vi "Initalise_Bike_Parameter.vi"(8 "Ts":dbl=8.0 format="%#_13g", 9 "Velocity":dbl=8.0 format="%#_13g") -> (0 "Other variables":T1, 1 "systems":T6 {"SysD"."Transport Delay" format="%.2f"; "SysD"."D" format="%#.2g"; "SysD"."C" format="%#.2g"; "SysD"."B" format="%#.2g"; "SysD"."A" format="%#.2g"; "SysD"."properties"."Sampling Time" format="%#.6p"; "SysD"."properties"."Output Delays" format="%.4f"; "SysD"."properties"."Input Delays" format="%.4f"; "sysDo"."Transport Delay" format="%.2f"; "sysDo"."D" format="%#.2g"; "sysDo"."C" format="%#.2g"; "sysDo"."B" format="%#.2g"; "sysDo"."A" format="%#.2g"; "sysDo"."properties"."Sampling Time" format="%#.6p"; "sysDo"."properties"."Output Delays" format="%.4f"; "sysDo"."properties"."Input Delays" format="%.4f"; "sysDi"."Transport Delay" format="%.2f"; "sysDi"."D" format="%#.2g"; "sysDi"."C" format="%#.2g"; "sysDi"."B" format="%#.2g"; "sysDi"."A" format="%#.2g"; "sysDi"."properties"."Sampling Time" format="%#.6p"; "sysDi"."properties"."Output Delays" format="%.4f"; "sysDi"."properties"."Input Delays" format="%.4f"; "sysDC"."transfer function(s)"."delay" format="%.4f"; "sysDC"."transfer function(s)"."Denominator" format="%#_3g"; "sysDC"."transfer function(s)"."Numerator" format="%#_3g"; "sysDC"."properties"."Sampling Time" format="%#.6p"; "sysDC"."properties"."Output Delays" format="%.4f"; "sysDC"."properties"."Input Delays" format="%.4f"})   [LabVIEW 2016]
uses:
  <vilib>/addons/Control Design/_Model Construction/Model Typedefs.llb/CD State Space Model (MIMO).ctl
  <vilib>/addons/Control Design/_Model Construction/Model Typedefs.llb/CD General Elements.ctl
  <vilib>/addons/Control Design/_Model Construction/Model Typedefs.llb/CD Transfer Function Model (MIMO).ctl
  <vilib>/addons/Control Design/_Model Construction/Model Typedefs.llb/CD Transfer Function Model (SISO).ctl
  <vilib>/imath/engines/lvmath2/RunTimeEngine/Managers/WorkSpace/UID Generator.vi
  <vilib>/imath/engines/lvmath2/RunTimeEngine/BuiltInFunctions/deg_to_rad/NIMS_deg_to_rad.vi
  <instcachedir>/0/NIMS_deg_to_rad_4A81D684CE8D4DD79924F5AB74D756E1.lvgen/NIMS_deg_to_rad_4A81D684CE8D4DD79924F5AB74D756E1_001.vi
  <vilib>/imath/engines/lvmath2/RunTimeEngine/BuiltInFunctions/inv/NIMS_inv(GM).vi
  <instcachedir>/0/NIMS_inv(GM)_A6DF8FE880224208AACFE4CF9F659502.lvgen/NIMS_inv(GM)_A6DF8FE880224208AACFE4CF9F659502_000.vi
  <vilib>/imath/engines/lvmath2/RunTimeEngine/ArithmeticOperatorToken/NIMS_ArithmeticOperator_multmx.vi
  <instcachedir>/0/NIMS_ArithmeticOperator_multmx_4A56FE5C615140CE835D4DB5891BF065.lvgen/NIMS_ArithmeticOperator_multmx_4A56FE5C615140CE835D4DB5891BF065_004.vi
  <vilib>/imath/engines/lvmath2/RunTimeEngine/ErrorHandling/NIMS_Create Error From Enums.vi
  <vilib>/imath/engines/lvmath2/RunTimeEngine/RowToken/NIMS_RowToken_M_M.vi
  <instcachedir>/0/NIMS_RowToken_M_M_968CDE3545E74ACDAEA4B48DE01EEECA.lvgen/NIMS_RowToken_M_M_968CDE3545E74ACDAEA4B48DE01EEECA_005.vi
  <instcachedir>/0/NIMS_RowToken_M_M_968CDE3545E74ACDAEA4B48DE01EEECA.lvgen/NIMS_RowToken_M_M_968CDE3545E74ACDAEA4B48DE01EEECA_004.vi
  <vilib>/imath/engines/lvmath2/RunTimeEngine/MatrixToken/NIMS_MatrixToken_M_M.vi
  <instcachedir>/0/NIMS_MatrixToken_M_M_DF273B0CC20F424BBF1EDA9F4E71C841.lvgen/NIMS_MatrixToken_M_M_DF273B0CC20F424BBF1EDA9F4E71C841_004.vi
  <vilib>/imath/engines/lvmath2/RunTimeEngine/ArithmeticOperatorToken/NIMS_ArithmeticOperator_multmx(M,CV).vi
  <instcachedir>/0/NIMS_ArithmeticOperator_multmx(M,CV)_EE734FC8520844C9A7CC1A67008668A3.lvgen/NIMS_ArithmeticOperator_multmx(M,CV)_EE734FC8520844C9A7CC1A67008668A3_002.vi
  <vilib>/imath/engines/lvmath2/RunTimeEngine/MatrixToken/NIMS_MatrixToken_SorCV_M.vi
  <instcachedir>/0/NIMS_MatrixToken_SorCV_M_667D6DA9EAAA4E73AD685CBB2779BCDB.lvgen/NIMS_MatrixToken_SorCV_M_667D6DA9EAAA4E73AD685CBB2779BCDB_000.vi
  <vilib>/imath/engines/lvmath2/RunTimeEngine/RowToken/NIMS_RowToken_CV_CV.vi
  <instcachedir>/0/NIMS_RowToken_CV_CV_5546A0B1CA2C4E49826F811B9C073FB0.lvgen/NIMS_RowToken_CV_CV_5546A0B1CA2C4E49826F811B9C073FB0_000.vi
  <vilib>/imathl/engines/lvmath/Functions/Error Handling/Create Error.vi
  <vilib>/imath/engines/lvmath/Plug In/Control Design/BuiltInFunctions/ss/NIMS_CD_ss(A,B,C,D).vi
  <vilib>/imath/engines/lvmath/Plug In/Control Design/BuiltInFunctions/c_to_d/NIMS_CD_c_to_d(SS,TS,STR,DBL).vi
  <vilib>/imath/engines/lvmath2/RunTimeEngine/RunTimeType/NIMS_RunTimeType_From StrictType (excl LVString).vi
  <instcachedir>/0/NIMS_RunTimeType_From StrictType (excl LVString)_BBF44FB49F834B71AF7A14CCEDF8BECD.lvgen/NIMS_RunTimeType_From StrictType (excl LVString)_BBF44FB49F834B71AF7A14CCEDF8BECD_031.vi
  <vilib>/imath/engines/lvmath2/RunTimeEngine/LocalVariableDefStatement/MC_LocalVariableDefStatement_Display.vi
  <vilib>/imath/engines/lvmath2/RunTimeEngine/ErrorHandling/NIMS_Error From Error Code.vi
  <vilib>/imath/engines/lvmath2/RunTimeEngine/IndexRead/NIMS M(S,S).vi
  <instcachedir>/0/NIMS M(S,S)_AC51E74150A542F7991B9634C66F3096.lvgen/NIMS M(S,S)_AC51E74150A542F7991B9634C66F3096_000.vi
  <instcachedir>/0/NIMS_RunTimeType_From StrictType (excl LVString)_BBF44FB49F834B71AF7A14CCEDF8BECD.lvgen/NIMS_RunTimeType_From StrictType (excl LVString)_BBF44FB49F834B71AF7A14CCEDF8BECD_000.vi
  <vilib>/imath/engines/lvmath/Plug In/Control Design/BuiltInFunctions/tf/NIMS_CD_tf(num,den,Ts).vi
  <vilib>/imath/engines/lvmath/Plug In/Control Design/BuiltInFunctions/c_to_d/NIMS_CD_c_to_d(TF,TS,STR,DBL).vi
  <vilib>/imath/engines/lvmath2/RunTimeEngine/Managers/SymbolTable/Clear UID.vi
  <vilib>/imath/engines/lvmath2/RunTimeEngine/NodeEndStatement/NIMS_NodeEndStatement_Output.vi
  <instcachedir>/0/NIMS_NodeEndStatement_Output_53EC0D466D134D7ABD903AC30B43404B.lvgen/NIMS_NodeEndStatement_Output_53EC0D466D134D7ABD903AC30B43404B_005.vi
  <instcachedir>/0/NIMS_NodeEndStatement_Output_53EC0D466D134D7ABD903AC30B43404B.lvgen/NIMS_NodeEndStatement_Output_53EC0D466D134D7ABD903AC30B43404B_011.vi
  <instcachedir>/0/NIMS_NodeEndStatement_Output_53EC0D466D134D7ABD903AC30B43404B.lvgen/NIMS_NodeEndStatement_Output_53EC0D466D134D7ABD903AC30B43404B_010.vi
  <instcachedir>/0/NIMS_NodeEndStatement_Output_53EC0D466D134D7ABD903AC30B43404B.lvgen/NIMS_NodeEndStatement_Output_53EC0D466D134D7ABD903AC30B43404B_001.vi
  <instcachedir>/0/NIMS_NodeEndStatement_Output_53EC0D466D134D7ABD903AC30B43404B.lvgen/NIMS_NodeEndStatement_Output_53EC0D466D134D7ABD903AC30B43404B_002.vi
  <vilib>/imath/engines/lvmath2/RunTimeEngine/ErrorHandling/NIMS_Finalize Error.vi
  <vilib>/imath/engines/lvmath2/RunTimeEngine/Managers/SymbolTable/NIMS_WorkSpace.lvlib
  <vilib>/addons/Control Design/_Model Construction/NI_LinSys_Model Typedefs.lvlib
panel:
  out "Lo":dbl[][](array[numeric])
  # "Inputs"
  # "Outputs"
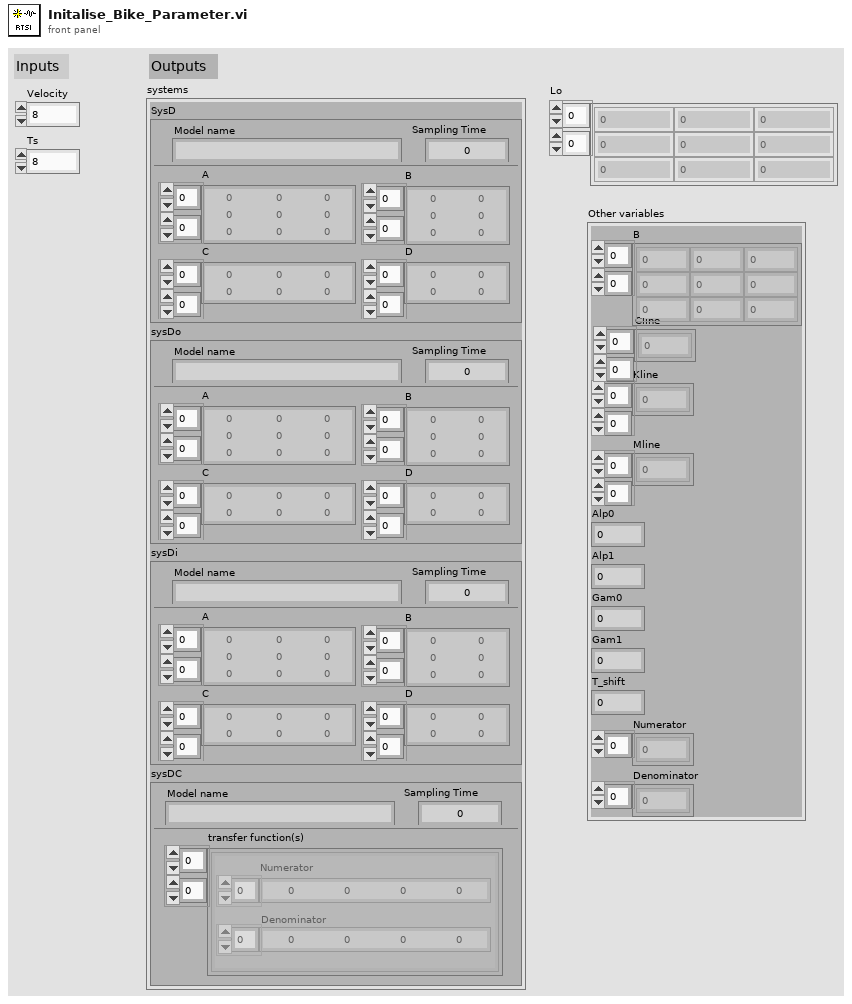
[diagram p1: front panel]
types:
  T1 = cluster{"B":dbl[][], "Cline":dbl[][], "Kline":dbl[][], "Mline":dbl[][], "Alp0":dbl, "Alp1":dbl, "Gam0":dbl, "Gam1":dbl, "T_shift":dbl, "Numerator":dbl[], "Denominator":dbl[]}
  T2 = typedef "NI_LinSys_Model Typedefs.lvlib/CD State Space Model (MIMO).ctl" = cluster{"properties":T3, "A":dbl[][], "B":dbl[][], "C":dbl[][], "D":dbl[][], "StateNames":string[], "Transport Delay":dbl[][]}
  T3 = typedef "NI_LinSys_Model Typedefs.lvlib/CD General Elements.ctl" = cluster{"Model name":string, "Input names":string[], "Output names":string[], "Input Delays":dbl[], "Output Delays":dbl[], "Sampling Time":dbl, "Notes":string}
  T4 = typedef "NI_LinSys_Model Typedefs.lvlib/CD Transfer Function Model (MIMO).ctl" = cluster{"properties":T3, "transfer function(s)":T5[][]}
  T5 = typedef "NI_LinSys_Model Typedefs.lvlib/CD Transfer Function Model (SISO).ctl" = cluster{"Numerator":dbl[], "Denominator":dbl[], "delay":dbl}
  T6 = cluster{"SysD":T2, "sysDo":T2, "sysDi":T2, "sysDC":T4}
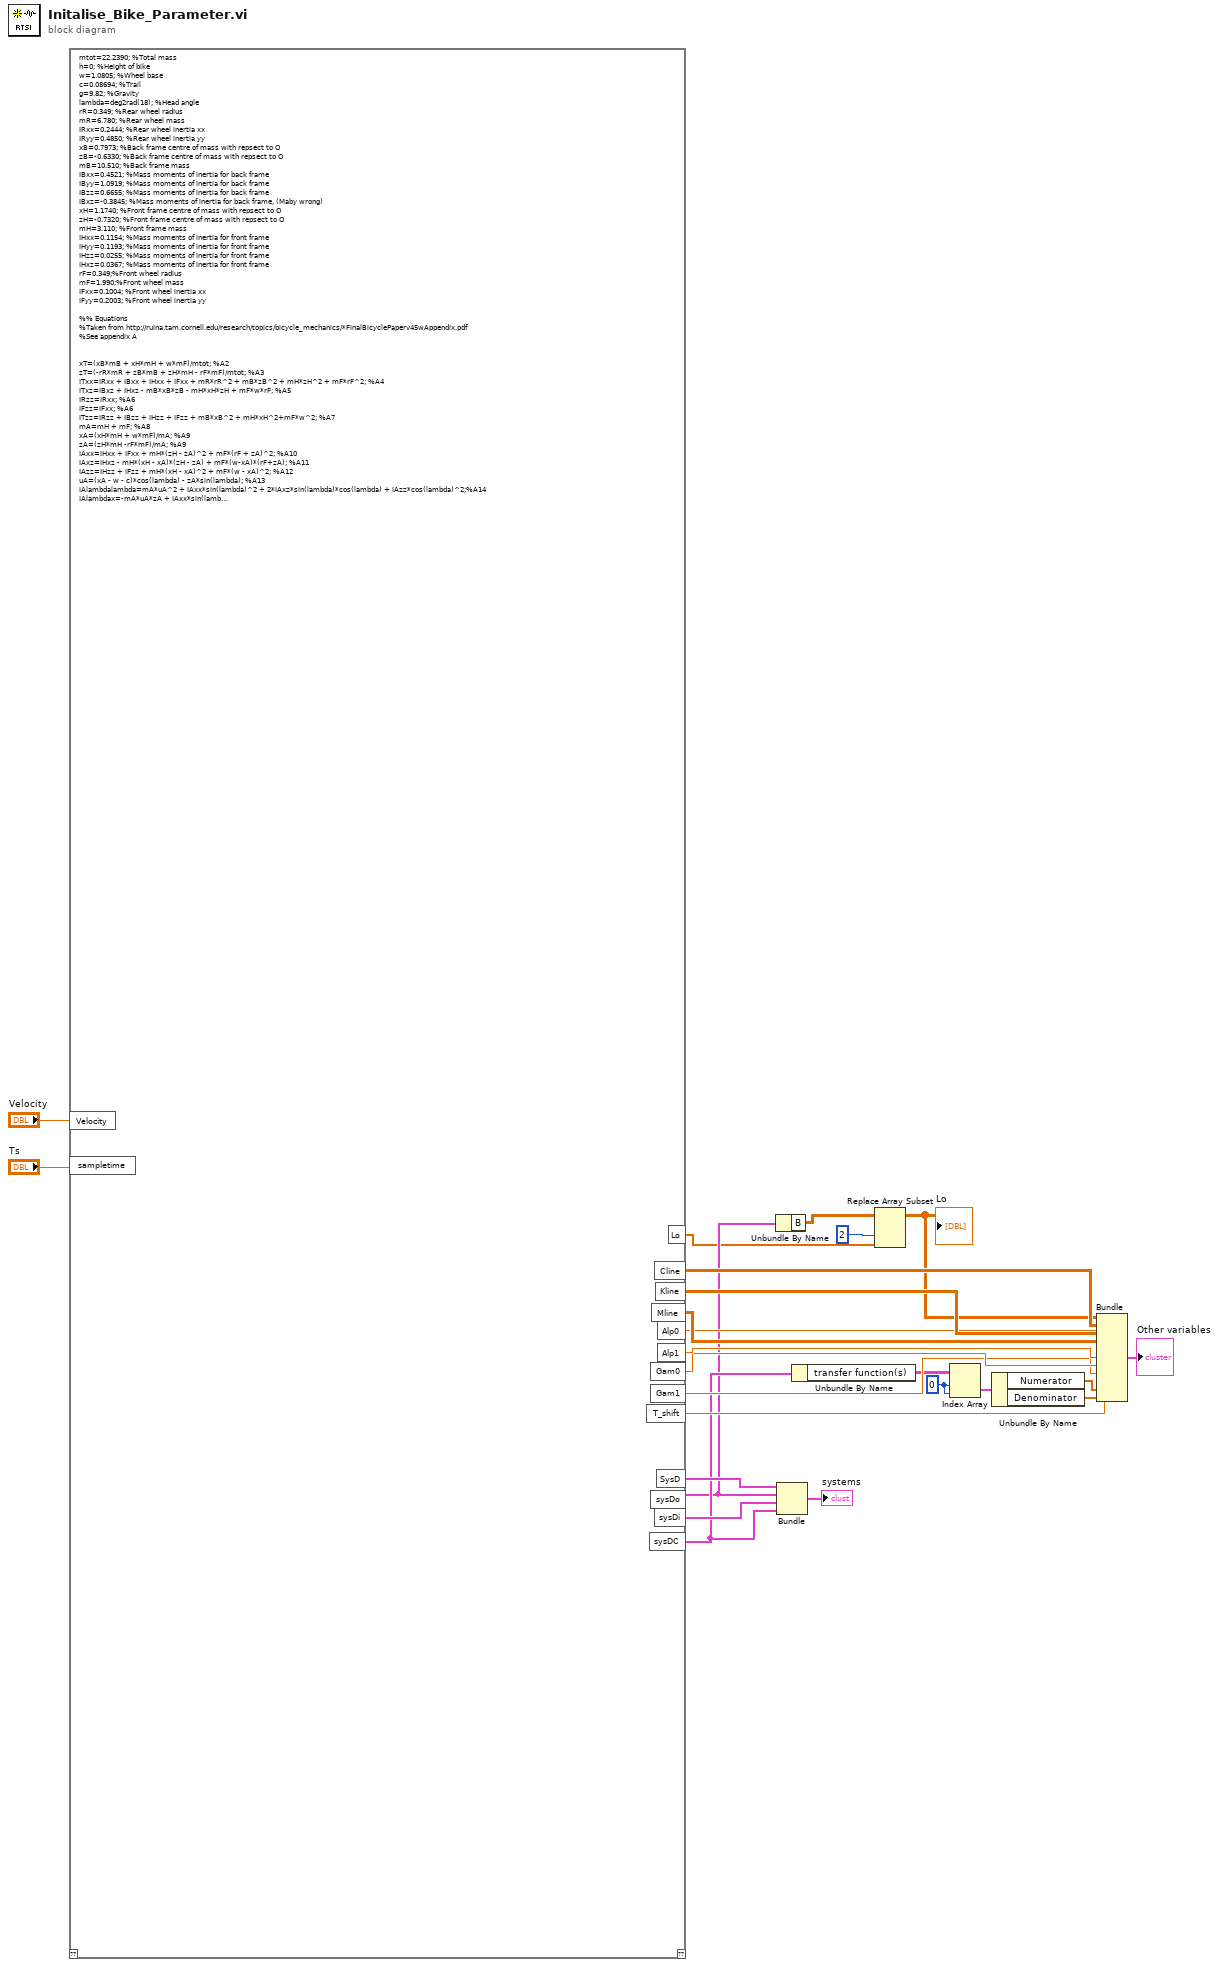
[diagram p0: block diagram]
diagram:
  w12 = 0 ("index (row)")
  n1 = mathscript code="mtot=22.2390; %Total mass\nh=0; %Height of bike\nw=1.0805; %Wheel base\nc=0.08694; %Trail\ng=9.82; %Gravity\nlambda=deg2rad(18); %Head angle\nrR=0.349; %Rear wheel radius\nmR=6.780; %Rear wheel mass\nIRxx=0.2444; %Rear wheel inertia xx\nIRyy=0.4850; %Rear wheel inertia yy\nxB=0.7973; %Back frame centre of mass with repsect to O\nzB=-0.6330; %Back frame centre of mass with repsect to O\nmB=10.510; %Back frame mass\nIBxx=0.4521; %Mass moments of inertia for back frame\nIByy=1.0919; %Mass moments of inertia for back frame\nIBzz=0.6655; %Mass moments of inertia for back frame\nIBxz=-0.3845; %Mass moments of inertia for back frame, (Maby wrong)\nxH=1.1740; %Front frame centre of mass with repsect to O\nzH=-0.7320; %Front frame centre of mass with repsect to O\nmH=3.110; %Front frame mass\nIHxx=0.1154; %Mass moments of inertia for front frame\nIHyy=0.1193; %Mass moments of inertia for front frame\nIHzz=0.0255; %Mass moments of inertia for front frame\nIHxz=0.0367; %Mass moments of inertia for front frame\nrF=0.349;%Front wheel radius\nmF=1.990;%Front wheel mass\nIFxx=0.1004; %Front wheel inertia xx\nIFyy=0.2003; %Front wheel inertia yy \n\n%% Equations\n%Taken from http://ruina.tam.cornell.edu/research/topics/bicycle_mechanics/*FinalBicyclePaperv45wAppendix.pdf\n%See appendix A\n\n\nxT=(xB*mB + xH*mH + w*mF)/mtot; %A2\nzT=(-rR*mR + zB*mB + zH*mH - rF*mF)/mtot; %A3\nITxx=IRxx + IBxx + IHxx + IFxx + mR*rR^2 + mB*zB^2 + mH*zH^2 + mF*rF^2; %A4\nITxz=IBxz + IHxz - mB*xB*zB - mH*xH*zH + mF*w*rF; %A5\nIRzz=IRxx; %A6\nIFzz=IFxx; %A6\nITzz=IRzz + IBzz + IHzz + IFzz + mB*xB^2 + mH*xH^2+mF*w^2; %A7\nmA=mH + mF; %A8\nxA=(xH*mH + w*mF)/mA; %A9\nzA=(zH*mH -rF*mF)/mA; %A9\nIAxx=IHxx + IFxx + mH*(zH - zA)^2 + mF*(rF + zA)^2; %A10\nIAxz=IHxz - mH*(xH - xA)*(zH - zA) + mF*(w-xA)*(rF+zA); %A11\nIAzz=IHzz + IFzz + mH*(xH - xA)^2 + mF*(w - xA)^2; %A12\nuA=(xA - w - c)*cos(lambda) - zA*sin(lambda); %A13\nIAlambdalambda=mA*uA^2 + IAxx*sin(lambda)^2 + 2*IAxz*sin(lambda)*cos(lambda) + IAzz*cos(lambda)^2;%A14\nIAlambdax=-mA*uA*zA + IAxx*sin(lambda) + IAxz*cos(lambda); %A15\nIAlambdaz=mA*uA*xA + IAxz*sin(lambda) + IAzz*cos(lambda); %A16\nmy=(c/w)*cos(lambda); %A17\nSR=IRyy/rR; %A18\nSF=IFyy/rF; %A18\nST=SR + SF; %A18\nSA=mA*uA + my*mtot*xT; %A19\nMfifi=ITxx; %A20\nMfidelta=IAlambdax + my*ITxz; %A20\nMdeltadelta=IAlambdalambda + 2*my*IAlambdaz + my^2*ITzz; %A20\nM=[Mfifi Mfidelta; Mfidelta Mdeltadelta]; %A21r\nK0fifi=mtot*zT; %A22\nK0fidelta=-SA; %A22\nK0deltadelta=-SA*sin(lambda); %A22\nK0=[K0fifi K0fidelta; K0fidelta K0deltadelta]; %A23\nK2fifi=0; %A24\nK2fidelta=((ST - mtot*zT)/w)*cos(lambda); %A24\nK2deltafi=0; %A24\nK2deltadelta=((SA + SF*sin(lambda))/w)*cos(lambda); %A24\nK2=[K2fifi K2fidelta; K2deltafi K2deltadelta]; %A25\nC1fifi=0; %A26\nC1fidelta=my*ST + SF*cos(lambda) + (ITxz/w)*cos(lambda) - my*mtot*zT; %A26\nC1deltafi=-(my*ST + SF*cos(lambda)); %A26\nC1deltadelta=(IAlambdaz/w)*cos(lambda) + my*(SA + (ITzz/w)*cos(lambda)); %A26\nC1=[C1fifi C1fidelta; C1deltafi C1deltadelta]; %A27\n %C=v*C1;\n Ts=sampletime;\n\n \n %%  Wipple model \n %A matrix\n v=Velocity/3.6;\n A1=[0 0; 0 0];\n A2=[1 0; 0 1];\n A3=-inv(M)*(g*K0+v^2*K2);\n A4=-inv(M)*v*C1;\n A=[A1, A2; A3, A4];\n \n %B matrix\n B=[[0; 0]; inv(M)*[0;1]]; \n %B1 matrix\n B1=[[0; 0]; inv(M)*[1;0]]; \n %C matrix\n C=[1 0 0 0; 0 1 0 0];\n %D matrix\n D=[0 0; 0 0];\n\nsys = ss(A, [B B1],C, D); \nSysD= c2d(sys,Ts)\n %% Lean angle control loop\n Cline=v*inv(M)*C1;\n Kline=inv(M)*(g*K0+v^2*K2);\n Mline=inv(M);\n\n%duty cycle constant\nKt=0.0273;\nKe=24/100;\nRm=0.33;\n\nDutyCycleTransform=0.009/((Mline(2,2)*Kt*Ke)/Rm); %duty cycle conversion \nT_shift=DutyCycleTransform; %torque conversion \n\n% Alpha and Gamma\nAlp1=4.367;\nAlp0=22.812\n\nGam1=38.538;\nGam0=448.438;\n\n \n%Outer control loop - stabilizing controller\n \nAo=[0 1 0; -Kline(1,1) -Cline(1,1) 1; 0 0 0]; %d \nBo=[0 0 1.557*10^3 ; 1 Mline(1,2) 5.386*10^5; 0 0 4.148*10^7]; \nCo=[1 0 0]; %f\nDo=[0 0 0]; %f\nLo=[2.097 257.5 1.346e+04]'\n \nsyso=ss(Ao,Bo,Co,Do);\nsysDo=c2d(syso, Ts);\n\n% modfi L gains \n%Lo=[2.097; 257.5 ;1.346e+04];\n%sysDo.B(:,3)=Lo;\n%Inner control loop - stabilizing controller\n \nAi=[0 1 0 0 0 0; -Kline(2,2) -Cline(2,2) 1 0 0 0; 0 0 0 1 0 0; 0 0 0 0 1 0; 0 0 0 0 0 1; 0 0 0 0 0 0];\nBi=[ 0 0 0 1.099*10^2; Mline(2,2) -Cline(2,1) -Kline(2,1) 4.693*10^3; 0  0  0 1.094*10^5;  0 0 0 0.22*10^5; 0 0 0 0.22*10^4; 0 0 0 0.3*10^2];\nCi=[1 0 0 0 0 0]; %f\nDi=[0 0 0 0]; %f\n \nsysi=ss(Ai,Bi,Ci,Di);\nsysDi=c2d(sysi, Ts);\n \n%% control structure\n \nsysC=tf(-1,[Cline(1,2) Kline(1,2)]);\n \nsysDC=c2d(sysC,Ts);"("Velocity"="Velocity", "sampletime"="Ts") -> ("Cline"=w24:dbl[][], "Kline"=w23:dbl[][], "Mline"=w22:dbl[][], "Alp0"=w21:dbl, "Alp1"=w20:dbl, "Gam0"=w19:dbl, "Gam1"=w18:dbl, "T_shift"=w17:dbl, "SysD"=w16:T2, "sysDo"=w6:T2, "sysDi"=w15:T2, "sysDC"=w11:T4, "Lo"=w4:dbl[])  [unwired: 1 in, 1 out]
  n2 = Unbundle By Name(w6) -> ("B"=w5:dbl[][])
  n3 = Bundle("SysD"=w16, "sysDo"=w6, "sysDi"=w15, "sysDC"=w11) -> (→"systems":T6)  [unwired: 1 in]
  n4 = Unbundle By Name ("Unbundle By Name 4")(w11) -> ("transfer function(s)"=w13:T5[][])
  n5 = Replace Array Subset(array=w5, new element=w4, index (col)=2 ("disabled index (col)")) -> (w2:dbl[][])  [unwired: 1 in]
  "Lo" <- w2
  n6 = Index Array(array=w13, index (row)=w12, index (col)=w12) -> (element=w10:T5)
  n7 = Unbundle By Name ("Unbundle By Name 5")(w10) -> ("Numerator"=w9:dbl[], "Denominator"=w8:dbl[])
  n8 = Bundle("B"=w2, "Cline"=w24, "Kline"=w23, "Mline"=w22, "Alp0"=w21, "Alp1"=w20, "Gam0"=w19, "Gam1"=w18, "T_shift"=w17, "Numerator"=w9, "Denominator"=w8) -> (→"Other variables":T1)  [unwired: 1 in]
